vi "KProp-Arg List to Table.vi"(0 "Rows in":T1[](array[typedef]), 5 "Args":string[](array[string]), 7 "type":string) -> (4 "Rows out":T1[](array[typedef]))   [LabVIEW 2020, in "KPropertyTable.xctl"]
uses:
  KPropertyTable.xctl
  RowData.ctl
  DataType.ctl
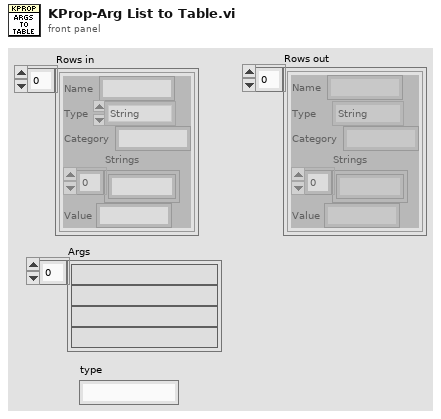
[diagram p1: front panel]
types:
  T1 = typedef "KPropertyTable.xctl/RowData.ctl" = cluster{"Name":string, "Type":T2, "Category":string, "Strings":string[], "Value":string}
  T2 = typedef "KPropertyTable.xctl/DataType.ctl" = enum16{"String", "Enum", "Int", "Double", "Boolean", "Ring", "Formula"}
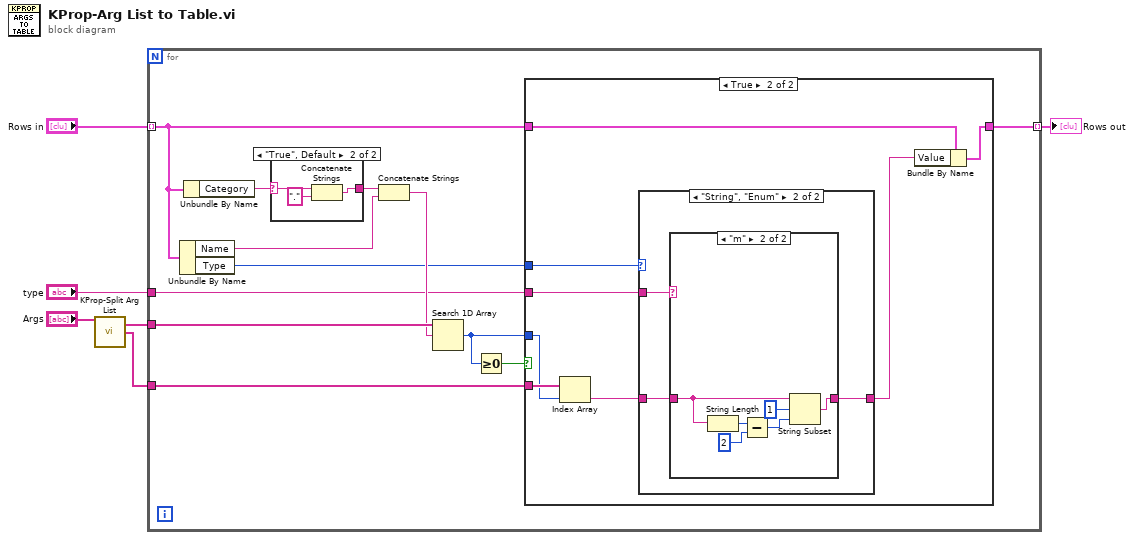
[diagram p0: block diagram]
diagram:
  n1 = call "KProp-Split Arg List.vi"("Args"="Args") -> ("Properties"=w3:string[], "Values"=w2:string[])  [unwired: 13 in]
  n2 = for {
    tunnel: "Rows in" -> [w10] mode=indexing
    tunnel: "type" -> [w7]
    tunnel: w3 -> [w15]
    tunnel: w2 -> [w11]
    tunnel: [w9] -> w1 mode=indexing
    n3 = Unbundle By Name(w10) -> ("Name"=w16:string, "Type"=w8:T2)
    n4 = Unbundle By Name(w10) -> ("Category"=w18:string)
    n5 = case shown="\"True\", Default" w18 {
      selector: w18 -> [w39 w42]
      tunnel: [w39 w41] -> w17
      frame "" {
      }
      frame "True", Default {
        n6 = Concatenate Strings(w42, "." ("string")) -> (w41:string)
      }
    }
    n7 = Concatenate Strings(w17, w16) -> (w14:string)
    n8 = Search 1D Array(1D array=w15, element=w14) -> (index of element=w12:i32)  [unwired: 1 in]
    n9 = Greater Or Equal To 0?(x=w12) -> (x >= 0?=w13:bool)
    n10 = case shown="True" w13 {
      tunnel: w12 -> [_ w26]
      tunnel: w11 -> [_ w27]
      tunnel: w10 -> [w19 w25]
      tunnel: [w19 w24] -> w9
      tunnel: w8 -> [_ w22]
      tunnel: w7 -> [_ w21]
      frame False {
      }
      frame True {
        n11 = Index Array(array=w27, index=w26) -> (element=w23:string)
        n12 = case shown="\"String\", \"Enum\"" w22 {
          tunnel: w23 -> [w28 w31]
          tunnel: w21 -> [_ w30]
          tunnel: [w28 w29] -> w20
          frame "Int", Default {
          }
          frame "String", "Enum" {
            n13 = case shown="\"m\"" w30 {
              tunnel: w31 -> [w32 w36]
              tunnel: [w32 w33] -> w29
              frame "vi", Default {
              }
              frame "m" {
                n14 = String Length(string=w36) -> (length=w37:i32)
                n15 = Subtract(x=w37, y=2) -> (x-y=w35:i32)
                n16 = String Subset(string=w36, offset (0)=1, length (rest)=w35) -> (substring=w33:string)
              }
            }
          }
        }
        n17 = Bundle By Name(cluster=w25, "Value"=w20) -> (w24:T1)
      }
    }
  }
  "Rows out" <- w1
